vi "LoopselFF - Copy (2).VI"() -> ()   [LabVIEW 2015]
panel:
  in  "?":enum32{"1", "2", "3"}(radio)=enum."3"
  in  "pos slope":u8=1
  in  "both slopes":u8
  in  "DAT in 10ns":u32
  out "FIFO overflow":bool
  in  "extTrig 0/1":u8
  in  "Start Read":bool
  in  "stop all":bool
  in  "Arm/Clear arry":bool
  in  "Slide":u32(slide)=89 scale=1.0..100.0
  in  "frequency[Hz]":u32
  in  "no.of samples (nos)":u32=100
  in  "exposuretime[ms]":dbl=1.0 format="%.3f"
  out "Signalverlaufgraph":u16[](graph)=[872, 298, 874, 874, 16384, 0, 88, 0, 6250, 6336, 6356, 6302, 6480, 6448, 6520, 6268, 6250, 6172, 6320, 6356, 6340, 6314, 6400, 6396, 6390, 6254, 6332, 6528, 6246, 6460, 6418, 6292, 6306, 6372, 6174, 6098, 6352, 6278, 6308, 6104, 6368, 6238, 6138, 6294, 6236, 6118, 6326, 6416, 6250, 6156, 6378, 6652, 6252, 6272, 6278, 6596, 6330, 6452, 6286, 6050, 6322, 6346, 6282, 6408, 6322, 6224, 6294, 6356, 6216, 6506, 6078, 6216, 6296, 6518, 6196, 6262, 6084, 6084, 6398, 6304, 6396, 6266, 6396, 6336, 6288, 6294, 6172, 6226, 6370, 6328, 6176, 6328, 6298, 6324, 6234, 6346, 6152, 6276, 6274, 6500, 6440, 6364, 6308, 6298, 6050, 6268, 6340, 6224, 6212, 6514, 6276, 6140, 6276, 6282, 6254, 6280, 6264, 6312, 6218, 6198, 6218, 6266, 6204, 6204, 6148, 6132, 6260, 6436, 6598, 6570, 6278, 6394, 6150, 6202, 6220, 5828, 938, 6280, 6372, 6392, 6306, 6268, 6520, 6306, 6254, 6260, 6268, 6328, 6564, 6510, 6364, 6504, 6442, 6126, 6438, 6288, 6448, 6248, 6306, 6262, 6138, 6504, 6324, 6266, 6392, 6504, 6204, 6238, 6388, 6336, 6428, 6298, 6410, 6344, 6472, 6292, 6598, 6646, 6164, 6276, 6366, 6262, 6284, 6336, 6306, 6270, 6288, 6404, 6500, 6414, 6550, 6316, 6308, 6324, 6376, 6320, 6428, 6604, 6360, 6494, 6284, 6548, 6506, 6004, 6368, 6320, 6112, 6328, 6330, 6282, 6418, 6460, 6416, 6276, 6392, 6120, 6278, 6338, 6362, 6396, 6440, 6294, 6266, 6282, 6204, 6084, 6168, 6262, 6460, 6304, 6278, 6130, 6356, 6220, 6456, 6372, 6286, 6286, 6314, 6396, 6520, 6298, 6276, 6358, 6424, 6446, 6218, 6280, 6286, 6156, 6254, 6330, 6148, 5992, 6356, 6432, 6362, 6264, 6356, 6132, 6424, 6264, 6304, 6310, 906, 6308, 6332, 6274, 6380, 6300, 6138, 6400, 6156, 6608, 6374, 6368, 6344, 6264, 6178, 6160, 6204, 6302, 6280, 6316, 6540, 6354, 6464, 6376, 6254, 6182, 6448, 6404, 6346, 6170, 6452, 6370, 6134, 6196, 6212, 6358, 6490, 6414, 6498, 6260, 6136, 6194, 6208, 6408, 6390, 6204, 6354, 6168, 6194, 6210, 6312, 6104, 6204, 6258, 5972, 6228, 6556, 6156, 6374, 6182, 6144, 6406, 6234, 6436, 6350, 6606, 6402, 6280, 6314, 6322, 6536, 6126, 6262, 6356, 6340, 6206, 6390, 6300, 6388, 6496, 6344, 6404, 6064, 6190, 6224, 6086, 6294, 6416, 6616, 6210, 6222, 6290, 6302, 6344, 6342, 6538, 6182, 6430, 6388, 6392, 6568, 6428, 6276, 6162, 6266, 6214, 6244, 6300, 6460, 6106, 6350, 6248, 6222, 6200, 6134, 6294, 6306, 6456, 6254, 6240, 6176, 6272, 6248, 6058, 6126, 6258, 6182, 6086, 952, 6158, 6338, 6366, 6342, 6240, 6278, 6232, 6436, 6406, 6712, 6808, 6514, 6872, 6674, 6338, 6464, 6362, 6502, 6368, 6528, 6208, 6646, 6386, 6346, 6268, 6400, 6534, 6382, 6580, 6484, 6332, 6552, 6658, 6702, 6384, 6326, 6162, 6158, 6488, 6558, 6512, 6064, 6446, 6464, 6220, 6480, 6426, 6300, 6380, 6432, 6320, 6338, 6114, 6166, 6382, 6514, 6494, 6724, 6400, 6430, 6348, 6428, 6556, 6658, 6452, 6328, 6392, 6474, 6624, 6366, 6544, 6322, 6270, 6296, 6514, 6162, 6494, 6454, 6384, 6408, 6884, 6092, 6268, 6430, 6168, 6370, 6586, 6886, 6378, 6448, 6594, 6636, 7158, 6684, 6152, 6322, 6606, 6174, 6420, 6890, 6718, 6498, 6658, 6848, 6442, 6476, 6546, 6498, 6510, 6538, 6594, 6294, 6188, 6262, 6504, 6488, 6530, 6774, 6568, 6210, 6400, 6488, 6312, 6348, 6396, 6594, 6478, 838, 5668, 5800, 5910, 6038, 5706, 6062, 6038, 6032, 6070, 5978, 5962, 5866, 5918, 6020, 5908, 6142, 5814, 6164, 5996, 6066, 6056, 5888, 5836, 5976, 5960, 5982, 5958, 5936, 6082, 5998, 6126, 6138, 6014, 5908, 6008, 6008, 6144, 5890, 5868, 6124, 5906, 6090, 5938, 6112, 5816, 6070, 5832, 5944, 5896, 5978, 5772, 6174, 5984, 5908, 5996, 5878, 5838, 5912, 5640, 5898, 6066, 5954, 5950, 6030, 5910, 6068, 5906, 5930, 5716, 5826, 5874, 6000, 6030, 5946, 5940, 5972, 5986, 6006, 6194, 6148, 6016, 6204, 6120, 6004, 6014, 6048, 5958, 6040, 6022, 6066, 5750, 6112, 6002, 5946, 5838, 5904, 5970, 5960, 6048, 6162, 5778, 6006, 5922, 5596, 5822, 6016, 5774, 5942, 6066, 6052, 6120, 6086, 5806, 5946, 5944, 6044, 6040, 5890, 5836, 5992, 6006, 6092, 6048, 6092, 5760, 5984, 6014, 754, 6228, 6258, 6250, 6038, 6154, 6212, 6090, 6372, 6210, 6230, 6424, 6104, 6274, 6142, 6442, 6210, 6346, 6124, 6084, 6132, 6184, 6410, 6304, 6520, 6308, 6148, 6288, 6200, 6168, 5906, 6204, 6150, 6326, 6342, 6500, 6258, 6416, 6284, 6042, 6306, 6212, 6198, 6194, 6208, 6124, 6302, 6340, 6446, 6450, 6136, 6154, 6356, 6260, 6280, 6324, 6068, 6188, 6374, 6240, 6382, 6158, 6238, 6248, 6304, 6404, 6302, 6332, 6376, 6446, 6180, 6376, 6394, 6108, 6188, 6264, 6356, 6222, 6330, 6556, 6488, 6252, 6250, 6320, 6366, 6174, 6302, 6186, 6352, 6304, 6114, 6442, 6434, 6380, 6090, 6166, 6236, 6258, 6402, 6474, 6560, 6124, 6348, 6326, 6458, 6596, 6306, 6474, 6210, 6264, 6110, 6184, 6322, 6276, 6406, 6198, 6118, 6220, 6358, 6436, 6226, 6332, 6066, 6464, 6376, 6280, 6510, 6646, 1056, 6342, 6432, 6686, 6982, 6786, 6638, 6990, 7128, 7102, 6674, 6566, 6604, 6840, 6692, 7112, 6996, 6752, 7124, 6770, 6790, 6668, 6984, 6798, 6856, 6782, 6840, 7026, 6896, 7140, 6896, 7356, 6998, 6546, 6714, 6636, 6900, 6508, 6650, 6668, 6962, 7038, 6792, 7122, 6708, 7028, 6852, 6842, 6650, 6948, 6840, 6816, 6740, 6542, 6796, 7062, 7458, 6808, 7060, 6482, 7038, 6952, 6806, 7080, 6854, 6988, 6918, 6470, 6462, 6974, 6776, 6808, 6776, 7012, 6724, 6808, 6684, 6870, 7296, 6968, 6892, 6932, 6982, 7114, 6482, 6494, 6460, 6560, 6266, 7098, 6838, 6756, 6888, 6890, 6586, 6852, 6534, 7204, 6768, 7560, 6806, 6696, 6862, 7040, 6932, 7012, 7242, 6846, 6742, 6444, 6778, 7344, 6906, 7244, 6932, 7018, 6832, 6840, 6718, 6960, 7412, 7116, 6720, 7128, 6960, 7046, 6708, 6882, 1002, 6244, 6478, 6598, 6940, 6830, 6960, 6928, 6528, 6790, 7396, 6890, 6698, 6506, 6844, 6910, 6614, 6854, 6672, 6570, 6556, 6352, 6376, 6392, 6556, 6694, 6652, 6884, 6838, 6720, 6610, 6340, 6764, 6920, 7096, 7180, 6848, 6494, 6632, 7008, 6670, 6706, 6954, 6926, 6658, 6708, 7046, 6464, 6576, 6434, 6194, 6592, 6888, 6988, 6934, 6754, 6590, 6726, 6468, 6518, 6920, 7220, 6878, 7124, 6810, 6854, 6598, 6686, 6850, 6858, 7134, 6952, 6576, 6288, 6434, 6680, 7176, 6876, 6924, 7524, 7220, 6672, 6702, 6682, 6830, 6478, 6410, 6748, 6970, 6334, 6456, 6388, 6796, 6838, 6796, 6490, 6678, 6344, 6552, 6486, 6902, 6986, 6684, 6906, 6616, 6798, 6668, 6852, 6752, 7190, 6336, 6662, 6784, 6904, 6572, 6600, 6728, 6796, 6858, 7170, 6900, 7116, 6846, 6660, 6950, 7076, 7114, 7306, 1024, 880, 868, 870, 868, 868, 868, 868, 868, 868, 868, 868, 868, 868, 868, 868, 868, 868, 868, 868, 868, 868, 868, 868, 868, 868, 868, 868, 868, 868, 868, 868, 868, 868, 868, 868, 868, 868, 868, 868, 868, 868, 868, 868, 868, 868, 868, 868, 868, 868, 868, 868, 868, 868, 868, 868]
  # "Start with run"
  # "Abort with ESC"
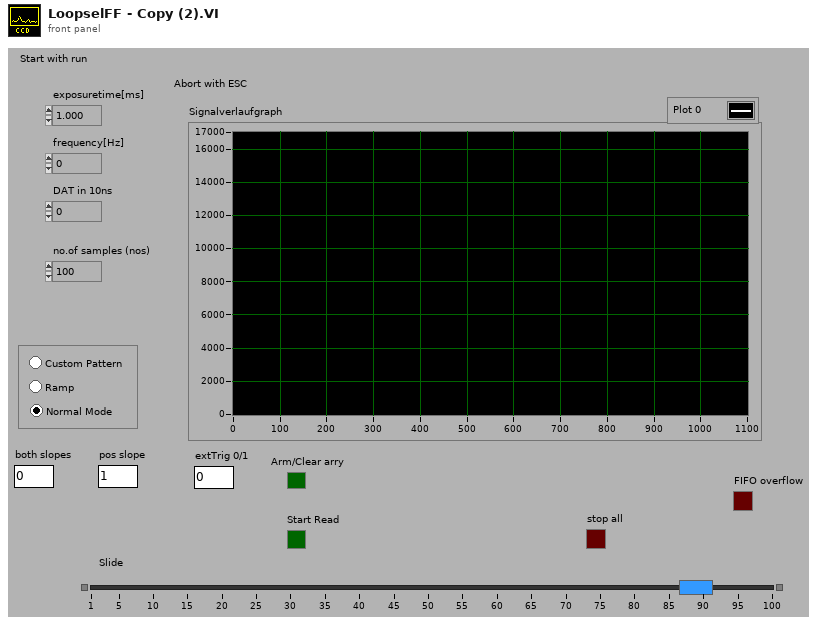
[diagram p1: front panel]
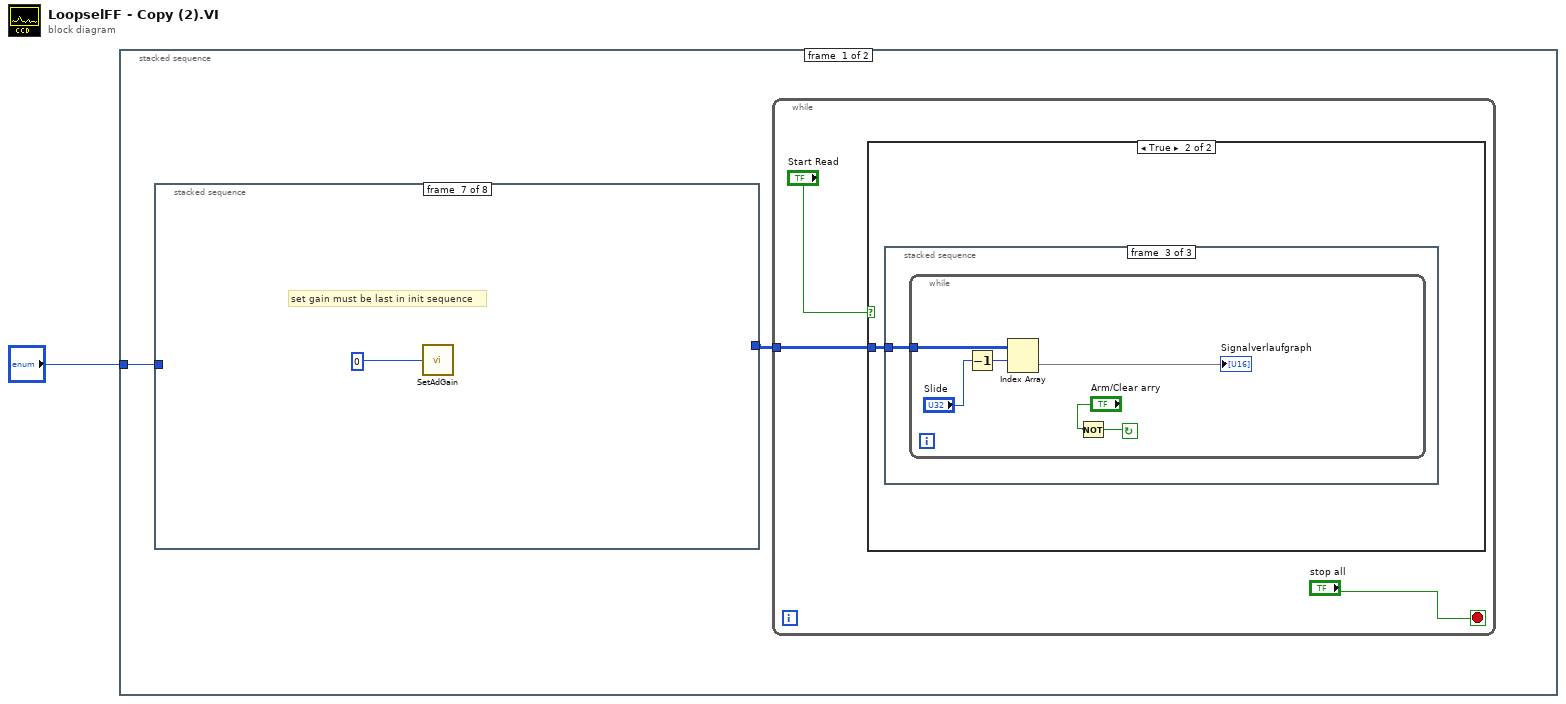
[diagram p0: block diagram]
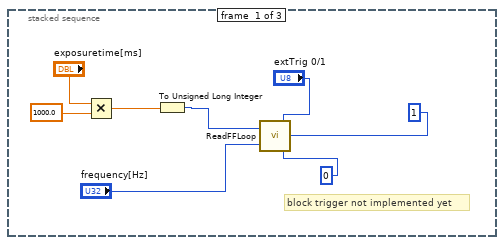
[diagram p3: hidden frame]
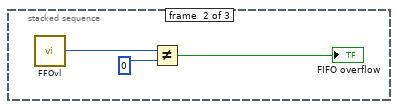
[diagram p4: hidden frame]
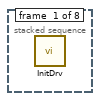
[diagram p5: hidden frame]
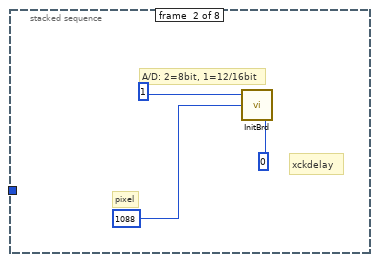
[diagram p6: hidden frame]
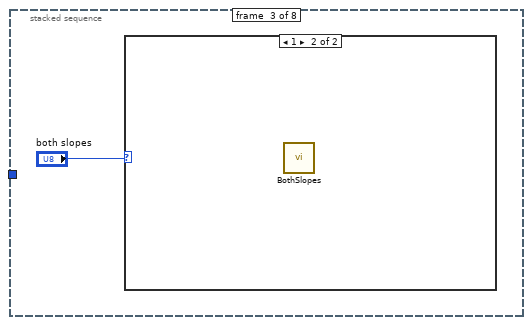
[diagram p7: hidden frame]
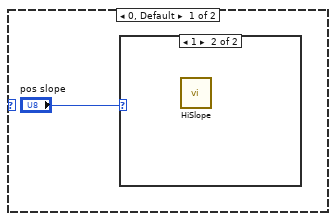
[diagram p8: hidden frame]
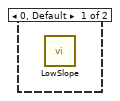
[diagram p9: hidden frame]
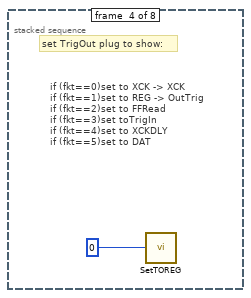
[diagram p10: hidden frame]
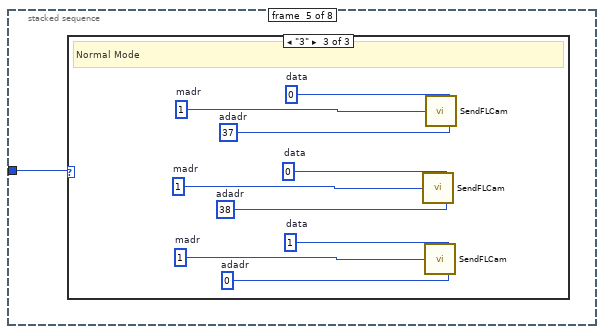
[diagram p11: hidden frame]
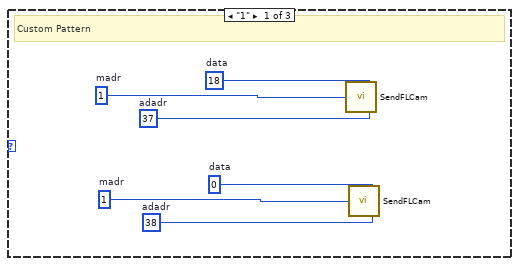
[diagram p12: hidden frame]
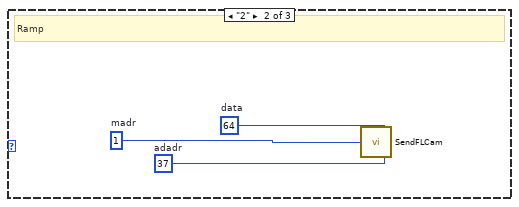
[diagram p13: hidden frame]
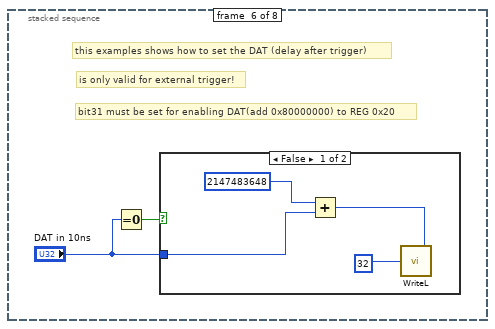
[diagram p14: hidden frame]
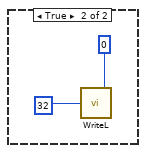
[diagram p15: hidden frame]
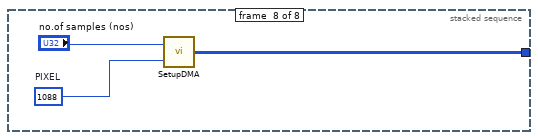
[diagram p16: hidden frame]
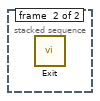
[diagram p17: hidden frame]
diagram:
  n1 = stacked-sequence {
    tunnel: "?" -> [w2 _]
    frame #0 {
      n2 = stacked-sequence {
        tunnel: [_ _ _ _ _ _ _ w62] -> w3
        tunnel: w2 -> [_ _ _ _ w32 _ _ _]
        frame #0 {
          n3 = call "InitDrv.vi"() -> ()  [unwired: 1 in]
        }
        frame #1 {
          # "pixel"
          # "xckdelay"
          # "A/D: 2=8bit, 1=12/16bit"
          n4 = call "InitBrd.vi"("xckdly"=u32 0, "pixel"=u32 1088, "flag816"=u32 1) -> ()  [unwired: 3 in]
        }
        frame #2 {
          n5 = case shown="1" "both slopes" {
            frame 0, Default {
              n6 = case shown="1" "pos slope" {
                frame 0, Default {
                  n7 = call "LowSlope.vi"() -> ()  [unwired: 1 in]
                }
                frame 1 {
                  n8 = call "HiSlope.vi"() -> ()  [unwired: 1 in]
                }
              }
            }
            frame 1 {
              n9 = call "BothSlopes.vi"() -> ()  [unwired: 1 in]
            }
          }
        }
        frame #3 {
          # "set TrigOut plug to show:"
          # "if (fkt==0)set to XCK -> XCK\nif (fkt==1)set to REG -> OutTrig\nif (fkt==2)set to FFRead\nif (fkt==3)set toTrigIn\nif (fkt==4)set to XCKDLY\nif (fkt==5)set to DAT"
          n10 = call "SetTOREG.vi"("fkt"=u8 0) -> ()
        }
        frame #4 {
          n11 = case shown="\"3\"" w32 {
            frame "1" {
              w33 = 0  # data
              w34 = 38  # adadr
              w35 = 1  # madr
              w36 = 18  # data
              w37 = 37  # adadr
              w38 = 1  # madr
              # "Custom Pattern"
              n12 = call "SendFLCam.vi"("madr"=w38, "data"=w36, "adadr"=w37) -> ()
              n13 = call "SendFLCam.vi"("madr"=w35, "data"=w33, "adadr"=w34) -> ()
            }
            frame "2" {
              w39 = 64  # data
              w40 = 37  # adadr
              w41 = 1  # madr
              # "Ramp"
              n14 = call "SendFLCam.vi"("madr"=w41, "data"=w39, "adadr"=w40) -> ()
            }
            frame "3" {
              w42 = 1  # data
              w44 = 0  # adadr
              w43 = 1  # madr
              w47 = 0  # data
              w46 = 38  # adadr
              w45 = 1  # madr
              w50 = 0  # data
              w49 = 37  # adadr
              w48 = 1  # madr
              # "Normal Mode"
              n15 = call "SendFLCam.vi"("madr"=w45, "data"=w47, "adadr"=w46) -> ()
              n16 = call "SendFLCam.vi"("madr"=w43, "data"=w42, "adadr"=w44) -> ()
              n17 = call "SendFLCam.vi"("madr"=w48, "data"=w50, "adadr"=w49) -> ()
            }
          }
        }
        frame #5 {
          # "bit31 must be set for enabling DAT(add 0x80000000) to REG 0x20"
          # "is only valid for external trigger!"
          # "this examples shows how to set the DAT (delay after trigger)"
          n18 = Equal To 0?(x="DAT in 10ns") -> (x = 0?=w52:bool)
          n19 = case shown="False" w52 {
            tunnel: "DAT in 10ns" -> [w53 _]
            frame False {
              n20 = Add(x=u32 2147483648, y=w53) -> (x+y=w56:u32)
              n21 = call "WriteL.vi"("val"=w56, "offset"=u32 32) -> ()
            }
            frame True {
              n22 = call "WriteL.vi"("val"=0, "offset"=u32 32) -> ()
            }
          }
        }
        frame #6 {
          # "set gain must be last in init sequence"
          n23 = call "SetAdGain.vi"("gain"=u8 0) -> ()  [unwired: 1 in]
        }
        frame #7 {
          w61 = u32 1088  # PIXEL
          n24 = call "SetupDMA.vi"("pixel"=w61, "nos"="no.of samples (nos)") -> ("Data Values"=w62:u16[][])
        }
      }
      n25 = while {
        tunnel: w3 -> [w5]
        stop <- "stop all" stop-if-true
        n26 = case shown="True" "Start Read" {
          tunnel: w5 -> [_ w7]
          frame False {
          }
          frame True {
            n27 = stacked-sequence {
              tunnel: w7 -> [_ _ w19]
              frame #0 {
                # "block trigger not implemented yet"
                n28 = Multiply(x="exposuretime[ms]", y=1000.0) -> (x*y=w15:dbl)
                n29 = To Unsigned Long Integer(number=w15) -> (unsigned 32bit integer=w12:u32)
                n30 = call "ReadFFLoop.vi"("exptus"=w12, "freq"="frequency[Hz]", "ExtTrig"="extTrig 0/1", "btrig_ch"=u32 1, "blocktrigger"=u8 0) -> ()
              }
              frame #1 {
                n31 = call "FFOvl.vi"() -> ("FFOvl"=w17:u8)  [unwired: 1 in]
                n32 = Not Equal?(x=w17, y=0) -> (x != y?=→"FIFO overflow":bool)
              }
              frame #2 {
                n33 = while {
                  tunnel: w19 -> [w21]
                  stop <- w25 continue-if-true
                  n34 = Decrement(x="Slide") -> (x-1=w23:u32)
                  n35 = Index Array(array=w21, index (row)=w23) -> (element=→"Signalverlaufgraph":u16[])  [unwired: 1 in]
                  n36 = Not(x="Arm/Clear arry") -> (.not. x?=w25:bool)
                }
              }
            }
          }
        }
      }
    }
    frame #1 {
      n37 = call "Exit.vi"() -> ()  [unwired: 1 in]
    }
  }
